vi "Graficadora.vi"() -> ()   [LabVIEW 2020]
panel:
  in  "stop":bool
  out "Alarma":bool
  out "Graficadora de Señal":dynamicdata(graph)
  in  "Temp":dbl(slide) scale=0.0..100.0
  in  "Lim":dbl
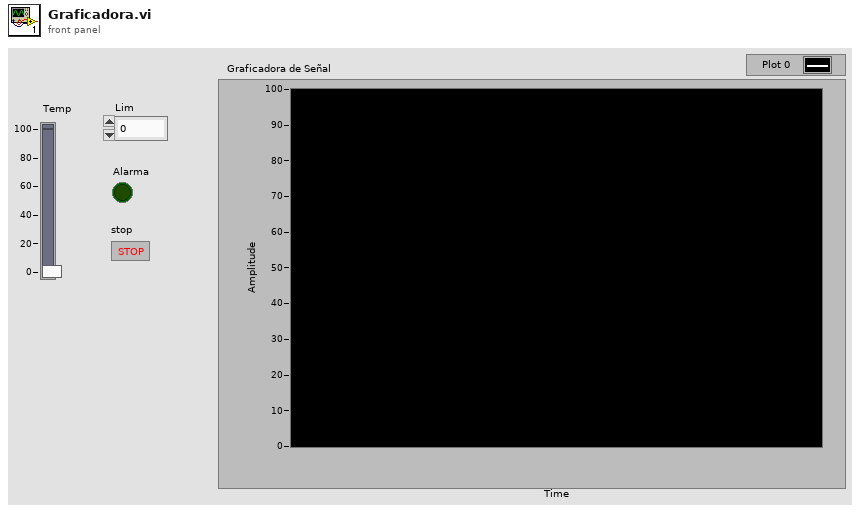
[diagram p1: front panel]
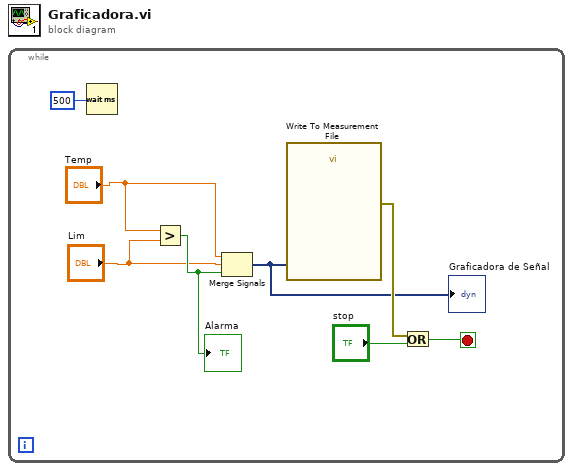
[diagram p0: block diagram]
diagram:
  n1 = while {
    stop <- w7 stop-if-true
    n2 = Wait (ms)(milliseconds to wait=500) -> ()  [unwired: 1 out]
    n3 = Greater?(x="Temp", y="Lim") -> (0:w4:bool)
    "Alarma" <- w4
    n4 = Merge Signals("Temp", "Lim", w4) -> (w6:dynamicdata)
    "Graficadora de Señal" <- w6
    n5 = call "Write To Measurement File"("Signals"=w6) -> ("error out"=w8:errorcluster)  [unwired: 16 in, 2 out]
    n6 = Or(x=w8, y="stop") -> (x .or. y?=w7:bool)
  }
